vi "Calculate rectangle pixels and lines.vi"(8 "No of Z planes":i32=1, 9 "Resolution multiplier":dbl=1.0, 10 "XY Coordinates (zero based)":i32[](array[numeric])) -> (1 "Number of lines (scaled)":dbl, 3 "Pixels in ROI":dbl, 4 "X pixels":dbl)   [LabVIEW 2020]
panel:
  # "X start\nY start\nX stop\nY stop"
  # "<--- Automatically switches to output the shortest dimension, assuming that rectangles longer on their Y axis are handled as vertical ROI, meaning that their X dimension becomes the number of lines/miniscans."
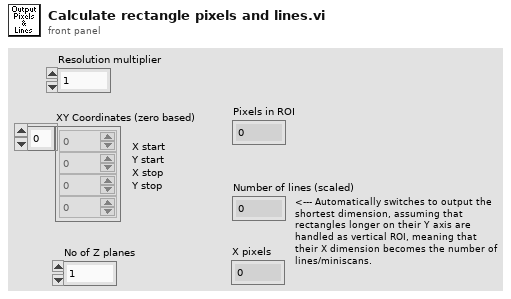
[diagram p1: front panel]
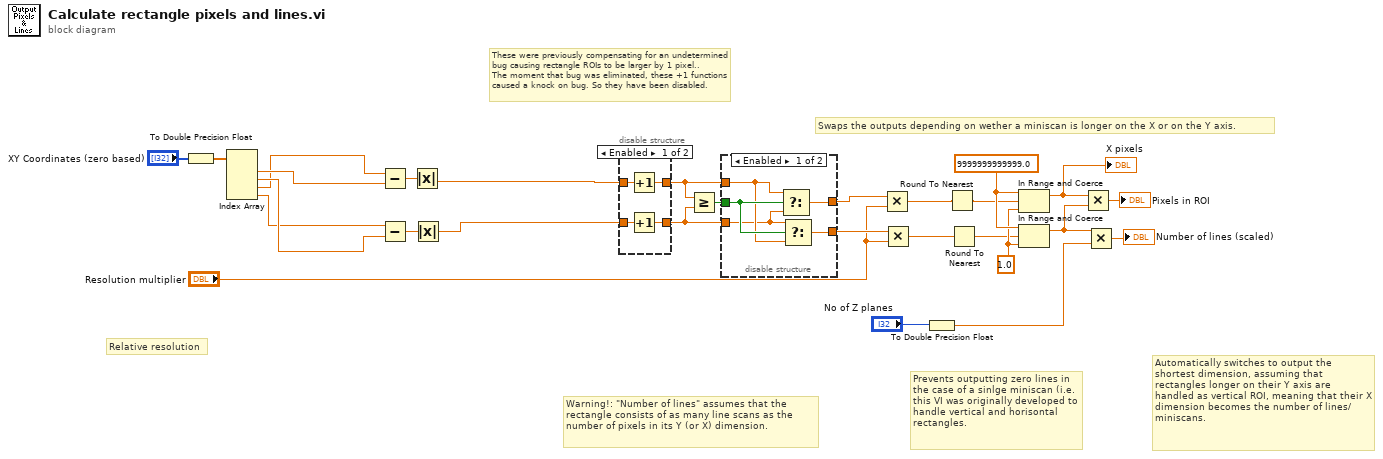
[diagram p0: block diagram]
diagram:
  w17 = 1.0 ("lower limit")
  w18 = 9999999999999.0 ("upper limit")
  # "Relative resolution"
  # "These were previously compensating for an undetermined bug causing rectangle ROIs to be larger by 1 pixel..\nThe moment that bug was eliminated, these +1 functions caused a knock on bug. So they have been disabled."
  # "Automatically switches to output the shortest dimension, assuming that rectangles longer on their Y axis are handled as vertical ROI, meaning that their X dimension becomes the number of lines/miniscans."
  # "Prevents outputting zero lines in the case of a sinlge miniscan (i.e. this VI was originally developed to handle vertical and horisontal rectangles."
  # "Warning!: \"Number of lines\" assumes that the rectangle consists of as many line scans as the number of pixels in its Y (or X) dimension."
  # "Swaps the outputs depending on wether a miniscan is longer on the X or on the Y axis."
  n1 = To Double Precision Float(number="XY Coordinates (zero based)") -> (double precision float=w20:dbl[])
  n2 = Index Array(array=w20) -> (element #1=w25:dbl, element #2=w24:dbl, element #3=w23:dbl, element #4=w22:dbl)  [unwired: 4 in]
  n3 = Subtract(x=w23, y=w25) -> (x-y=w27:dbl)
  n4 = Subtract(x=w22, y=w24) -> (x-y=w28:dbl)
  n5 = Absolute Value(x=w27) -> (abs(x)=w8:dbl)
  n6 = Absolute Value(x=w28) -> (abs(x)=w9:dbl)
  n7 = disable-structure shown="Enabled" {
    disable-tunnel: w8 -> [w32 w34]
    disable-tunnel: w9 -> [w31 w33]
    disable-tunnel: [w30 w34] -> w16
    disable-tunnel: [w29 w33] -> w15
    frame Enabled {
      n8 = Increment(x=w32) -> (x+1=w30:dbl)
      n9 = Increment(x=w31) -> (x+1=w29:dbl)
    }
    frame Disabled {
    }
  }
  n10 = Greater Or Equal?(x=w16, y=w15) -> (x >= y?=w26:bool)
  n11 = disable-structure shown="Enabled" {
    disable-tunnel: w26 -> [w39 _]
    disable-tunnel: [w38 w41] -> w7
    disable-tunnel: [w37 w40] -> w6
    disable-tunnel: w16 -> [w36 w40]
    disable-tunnel: w15 -> [w35 w41]
    frame Enabled {
      n12 = Select(t=w36, s=w39, f=w35) -> (s? t:f=w38:dbl)
      n13 = Select(t=w35, s=w39, f=w36) -> (s? t:f=w37:dbl)
    }
    frame Disabled {
    }
  }
  n14 = Multiply(x=w7, y="Resolution multiplier") -> (x*y=w4:dbl)
  n15 = Multiply(x=w6, y="Resolution multiplier") -> (x*y=w2:dbl)
  n16 = To Double Precision Float(number="No of Z planes") -> (double precision float=w11:dbl)
  n17 = Round To Nearest(number=w4) -> (nearest integer value=w3:dbl)
  n18 = Round To Nearest(number=w2) -> (nearest integer value=w1:dbl)
  n19 = In Range and Coerce(upper limit=w18, x=w3, lower limit=w17) -> (coerced(x)=w19:dbl)  [unwired: 1 out]
  "X pixels" <- w19
  n20 = In Range and Coerce(upper limit=w18, x=w1, lower limit=w17) -> (coerced(x)=w12:dbl)  [unwired: 1 out]
  n21 = Multiply(x=w19, y=w12) -> (x*y=→"Pixels in ROI":dbl)
  n22 = Multiply(x=w12, y=w11) -> (x*y=→"Number of lines (scaled)":dbl)
